vi "Show A3 Dataoutput.vi"() -> ()   [LabVIEW 2018]
uses:
  <vilib>/myRIO/Instrument Drivers/Onboard IO/UART/typedef/VISA Configuration.ctl
  <vilib>/Instr/_visa.llb/VISA Configure Serial Port (Instr).vi
  <vilib>/myRIO/Instrument Drivers/Onboard IO/UART/UART.lvlib
panel:
  in  "stop":bool
  out "Latest String A3":string
  in  "VISA Refnum in":refnum<visa-resource-name>
  in  "error in (no error)":errorcluster
  out "error out":errorcluster
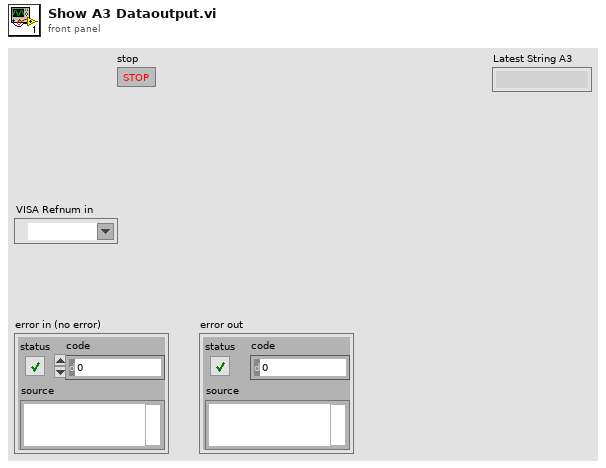
[diagram p1: front panel]
types:
  T1 = typedef "UART.lvlib/VISA Configuration.ctl" = cluster{"baud rate (9600)":u32, "data bits (8)":u16, "parity (0:none)":enum16{"None", "Odd", "Even", "Mark", "Space"}, "stop bits (10: 1 bit)":u16, "flow control (0:none)":u16, "termination char\n(0xA = '\\n' = LF) ":u8, "Enable Termination\nChar (T)":bool, "timeout (10sec)":u32}
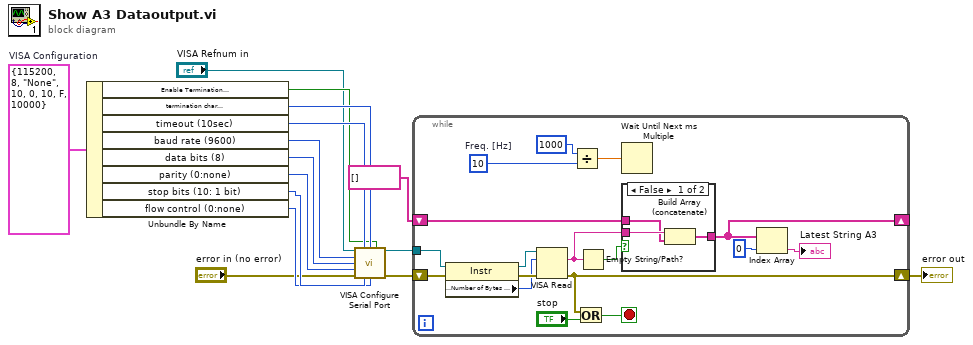
[diagram p0: block diagram]
diagram:
  w5 = T1 {"baud rate (9600)"=115200, "data bits (8)"=8, "parity (0:none)"=enum."None", "stop bits (10: 1 bit)"=10, "flow control (0:none)"=0, "termination char\n(0xA = '\\n' = LF) "=10, "Enable Termination\nChar (T)"=FALSE, "timeout (10sec)"=10000}  # VISA Configuration
  n1 = Unbundle By Name(w5) -> ("Enable Termination\nChar (T)"=w8:bool, "termination char\n(0xA = '\\n' = LF)"=w9:u8, "timeout (10sec)"=w10:u32, "baud rate (9600)"=w15:u32, "data bits (8)"=w14:u16, "parity (0:none)"=w13:enum16{"None", "Odd", "Even", "Mark", "Space"}, "stop bits (10: 1 bit)"=w12:u16, "flow control (0:none)"=w11:u16)
  n2 = call-poly "VISA Configure Serial Port"("VISA resource name"="VISA Refnum in", "timeout (10sec)"=w10, "termination char\n(0xA = '\\n' = LF)"=w9, "Enable Termination\nChar (T)"=w8, "baud rate (9600)"=w15, "data bits (8)"=w14, "parity (0:none)"=w13, "error in (no error)"="error in (no error)", "stop bits (10: 1 bit)"=w12, "flow control (0:none)"=w11) -> ("VISA resource name out"=w3:refnum<visa-resource-name>, "error out"=w2:errorcluster)  [unwired: 4 in]
  n3 = while {
    tunnel: w3 -> [w32]
    shift-right: [w20] -> w7
    shift-left: w2 -> [w30]
    shift-right: [w24] -> _
    shift-left: string[] [] -> [w25]
    stop <- w21 stop-if-true
    w16 = 10  # Freq. [Hz]
    n4 = property class="Instr"(reference=w32, error in=w30) -> (reference out=w31:refnum<visa-resource-name>, error out=w29:errorcluster, "Serial Settings:Number of Bytes at Serial Port"=w28:u32)
    n5 = VISA Read(VISA resource name=w31, byte count=w28, error in (no error)=w29) -> (read buffer=w26:string, error out=w20:errorcluster)  [unwired: 2 out]
    n6 = Divide(x=1000, y=w16) -> (x/y=w17:dbl)
    n7 = Or(x=w20, y="stop") -> (x .or. y?=w21:bool)
    n8 = Empty String/Path?(string/path=w26) -> (empty?=w27:bool)
    n9 = Wait Until Next ms Multiple(millisecond multiple=w17) -> ()  [unwired: 1 out]
    n10 = case shown="False" w27 {
      tunnel: w26 -> [w35 _]
      tunnel: [w34 w36] -> w24
      tunnel: w25 -> [w33 w36]
      frame False {
        n11 = Build Array (concatenate)(w35, w33) -> (w34:string[])
      }
      frame True {
      }
    }
    n12 = Index Array(array=w24, index=0) -> (element=→"Latest String A3":string)
  }
  "error out" <- w7
